vi "Send ERROR.vi"(8 "error in (no error)":errorcluster, 10 "Error Request":T1={"WAMP Error"={"Details"="{}", "ArgumentKw Payload"="", "Error?"=FALSE, "Error URI"="", "Arguments Payload"=""}, "Message Type"=0, "Request ID"=0} {"Message Type" items=["HELLO"=1, "WELCOME"=2, "ABORT"=3, "GOODBYE"=6, "ERROR"=8, "PUBLISH"=16, "PUBLISHED"=17, "SUBSCRIBE"=32, "SUBSCRIBED"=33, "UNSUBSCRIBE"=34, "UNSUBSCRIBED"=35, "EVENT"=36, "CALL"=48, "RESULT"=59, "REGISTER"=64, "REGISTERED"=65, "UNREGISTER"=66, "UNREGISTERED"=67, "INVOCATION"=68, "YIELD"=70]}, 11 "WAMP Client in":refnum<class "WAMP Client.lvclass">) -> (0 "error out":errorcluster, 3 "WAMP Client out":refnum<class "WAMP Client.lvclass">)   [LabVIEW 2020, in "wamplv.lvlib" / "WAMP Client.lvclass"]
uses:
  WAMP Client.lvclass
  API/TypeDefs/WAMP error.ctl
  TypeDef/WAMP Message Codes.ctl
  TypeDef/Error Request.ctl
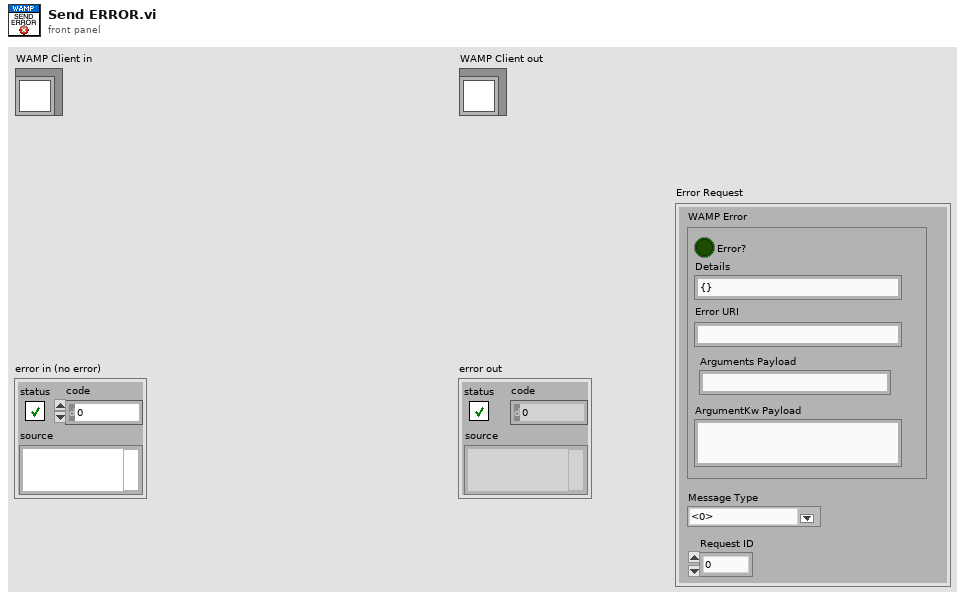
[diagram p1: front panel]
types:
  T1 = typedef "wamplv.lvlib/WAMP Client.lvclass/Error Request.ctl" = cluster{"WAMP Error":T2, "Message Type":T3, "Request ID":u64}
  T2 = typedef "wamplv.lvlib/WAMP Client.lvclass/WAMP error.ctl" = cluster{"Details":string, "ArgumentKw Payload":string, "Error?":bool, "Error URI":string, "Arguments Payload":string}
  T3 = typedef "wamplv.lvlib/WAMP Client.lvclass/WAMP Message Codes.ctl" = u16
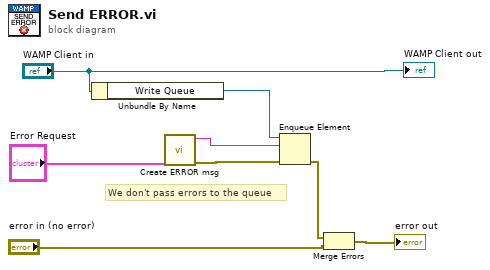
[diagram p0: block diagram]
diagram:
  # "We don't pass errors to the queue"
  n1 = Unbundle By Name("WAMP Client in") -> ("Write Queue"=w5:refnum<queue>)
  n2 = call "Create ERROR msg.vi"("Error Request"="Error Request") -> ("error out"=w6:errorcluster, "String"=w7:string)  [unwired: 9 in]
  n3 = Enqueue Element(queue=w5, element=w7, error in (no error)=w6) -> (error out=w4:errorcluster)  [unwired: 1 in, 2 out]
  n4 = Merge Errors(w4, "error in (no error)") -> (→"error out":errorcluster)
  "WAMP Client out" <- "WAMP Client in"
